vi "2.vi"() -> ()   [LabVIEW 2017]
uses:
  <userlib>/_OpenG.lib/string/string.llb/Trim Whitespace (String Array)__ogtk.vi
  <userlib>/_OpenG.lib/array/array.llb/Filter 1D Array with Scalar (String)__ogtk.vi
panel:
  out "error in (no error) (dup)":errorcluster
  in  "error in (no error)":errorcluster
  out "The Count":i32
  in  "String":string
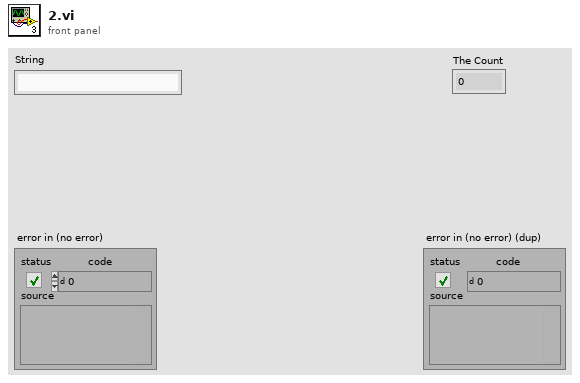
[diagram p1: front panel]
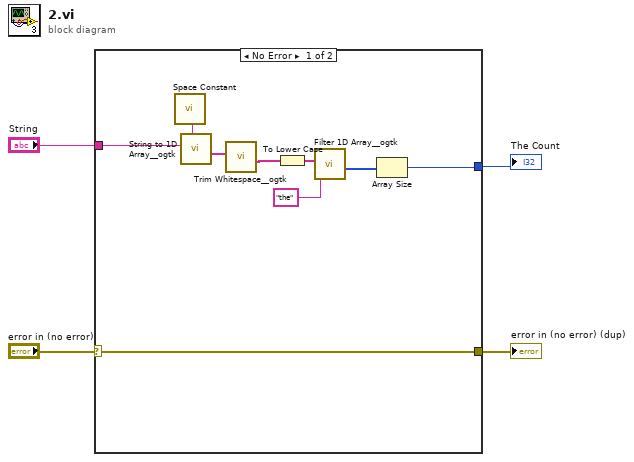
[diagram p0: block diagram]
diagram:
  n1 = case shown="No Error" "error in (no error)" {
    selector: "error in (no error)" -> [w13 w14]
    tunnel: [w13 w14] -> w3
    tunnel: "String" -> [w12 _]
    tunnel: [w5 _] -> w1
    frame No Error {
      n2 = call <vilib>:"Space Constant.vi"() -> ("String"=w11:string)
      n3 = call <userlib>:"String to 1D Array__ogtk.vi"("delimiter (Tab)"=w11, "string"=w12) -> ("Array of Strings"=w10:string[])  [unwired: 9 in]
      n4 = call-poly <userlib>:"Trim Whitespace__ogtk.vi"("String in"=w10) -> ("String out"=w9:string[])  [unwired: 6 in]
      n5 = To Lower Case(string=w9) -> (all lower case string=w8:string[])
      n6 = call-poly <userlib>:"Filter 1D Array__ogtk.vi"("items to filter"="the", "array"=w8) -> ("filtered item indices"=w6:i32[])  [unwired: 4 in, 1 out]
      n7 = Array Size(array=w6) -> (size(s)=w5:i32)
    }
    frame Error {
    }
  }
  "The Count" <- w1
  "error in (no error) (dup)" <- w3
